vi "testDBL2.vi"() -> ()   [LabVIEW 2026]
panel:
  out "Waveform Graph":dbl[](graph)
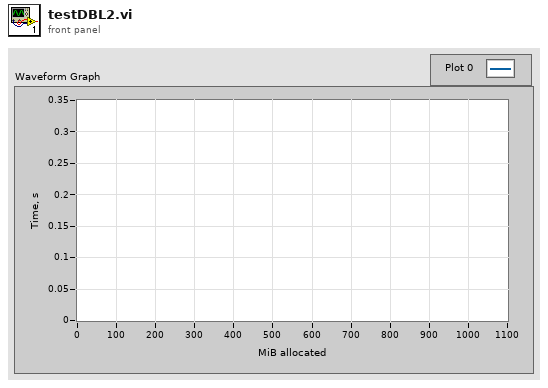
[diagram p1: front panel]
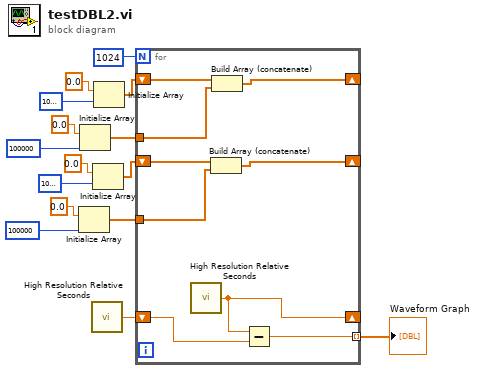
[diagram p0: block diagram]
diagram:
  n1 = Initialize Array(0.0 ("element"), 100000 ("dimension size")) -> (w7:dbl[])
  n2 = Initialize Array(0.0 ("element"), 100000 ("dimension size")) -> (w6:dbl[])
  n3 = call <vilib>:"High Resolution Relative Seconds.vi"() -> ("relative seconds"=w11:dbl)
  n4 = Initialize Array(0.0 ("element"), 1048576 ("dimension size")) -> (w13:dbl[])
  n5 = Initialize Array(0.0 ("element"), 1048576 ("dimension size")) -> (w3:dbl[])
  n6 = for {
    N: 1024 -> [_]
    shift-right: [w23] -> _
    shift-left: w13 -> [w24]
    shift-right: [w20] -> _
    shift-left: w11 -> [w22]
    tunnel: [w21] -> w10 mode=indexing
    tunnel: w7 -> [w19]
    shift-right: [w17] -> _
    shift-left: w3 -> [w16]
    tunnel: w6 -> [w18]
    n7 = call <vilib>:"High Resolution Relative Seconds.vi"() -> ("relative seconds"=w20:dbl)
    n8 = Build Array (concatenate)(w24, w19) -> (w23:dbl[])
    n9 = Build Array (concatenate)(w16, w18) -> (w17:dbl[])
    n10 = Subtract(x=w20, y=w22) -> (x-y=w21:dbl)
  }
  "Waveform Graph" <- w10
